vi "TEST Resize to Largest Decoration.vi"() -> ()   [LabVIEW 2011]
panel:
  in  "stop":bool
  out "Waveform Chart":dbl(graph)
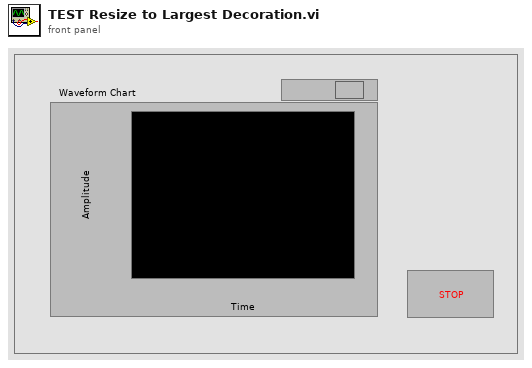
[diagram p1: front panel]
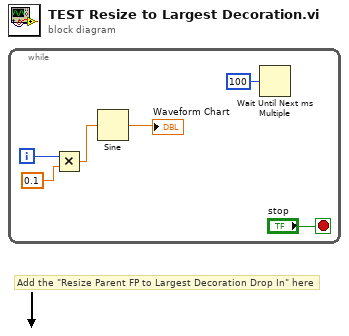
[diagram p0: block diagram]
diagram:
  # "Add the \"Resize Parent FP to Largest Decoration Drop In\" here"
  n1 = while {
    i -> [w3]
    stop <- "stop" stop-if-true
    n2 = Multiply(x=w3, y=0.1) -> (x*y=w1:dbl)
    n3 = Sine(x=w1) -> (sin(x)=→"Waveform Chart":dbl)
    n4 = Wait Until Next ms Multiple(millisecond multiple=u32 100) -> ()  [unwired: 1 out]
  }
